vi "LIVE+PSM+SAVING_modified.vi"() -> ()   [LabVIEW 2020]
uses:
  C:/Users/Hannah/Documents/GitHub/pan-ASLM/LabVIEW camera PVCam/Dependencies/PVCamNET.dll
  Dependencies/PVCamNET.dll
panel:
  out "Min  2":u32
  out "Max 2":u32
  out "RawImageData 3":u16[](array[numeric])
  out "SavingPath":string="C:\\Users\\Hannah\\Downloads\\Parameters\\"
  in  "Path":path=path "C:/Users/Hannah/Downloads/Parameters"
  in  "exposure resolution":enum16{"milliseconds", "Microseconds"}(ring)
  out "Saving":bool
  out "Capturing":bool
  in  "seq_save":bool
  in  "seq_start":bool
  in  "FramesToCapture":u16
  in  "Full CCD Height":u16=3200
  in  "Full CCD Width":u16=3200
  in  "Full CCD":bool
  in  "Get ROI":bool
  in  "Height":u16=3192
  in  "Y":u16=4
  in  "Width":u16=416
  in  "X":u16=1452
  out "Trigger Mode":i32=2304
  in  "Trigger In Behaviour":string(combo)="Internal Trigger"
  out "Exp. out":i32
  in  "Trigger Out Behaviour":string(combo)="First Row"
  out "Boolean":bool
  in  "Scan Direction Reset":bool
  out "Scan Line Time":dbl=7063.0 format="%#_14g"
  in  "Scan Width":dbl
  in  "Scan Line Delay":dbl=2.0
  in  "Scan Direction":string(combo)="Down"
  in  "Scan Mode":string(combo)="Auto"
  in  "Exposure Time":dbl=10.0
  in  "Live":bool
  in  "Camera Status":bool
  in  "Uninit":bool
  in  "Live stop":bool
  in  "Live start":bool
  in  "Open":bool
  # "Do not press the red LabVIEW circular button – this will not properly close the camera."
  # "Description:\nThis interface can be used for both live imaging\nand sequence acquisition.\n\nSteps to run:\n1. Click the \"Run\" arrow\n2. Click \"Open\"\n3. Add desired parameters\n\nTo run live imaging: click \"Live Start\". If\nparameters need to be changed while imaging,\nfirst click \"Live Stop\" and then change\nparameters before starting again.\n\nTo execute sequence acquisition: click\n\"Sequence Start\". AFTER sequence has been\ncompleted (signified by the \"Capturing\" light\nturning off), click \"Sequence Save\" to save\nimages to desired folder.\n\n4. Click \"Close\" after finished imaging"
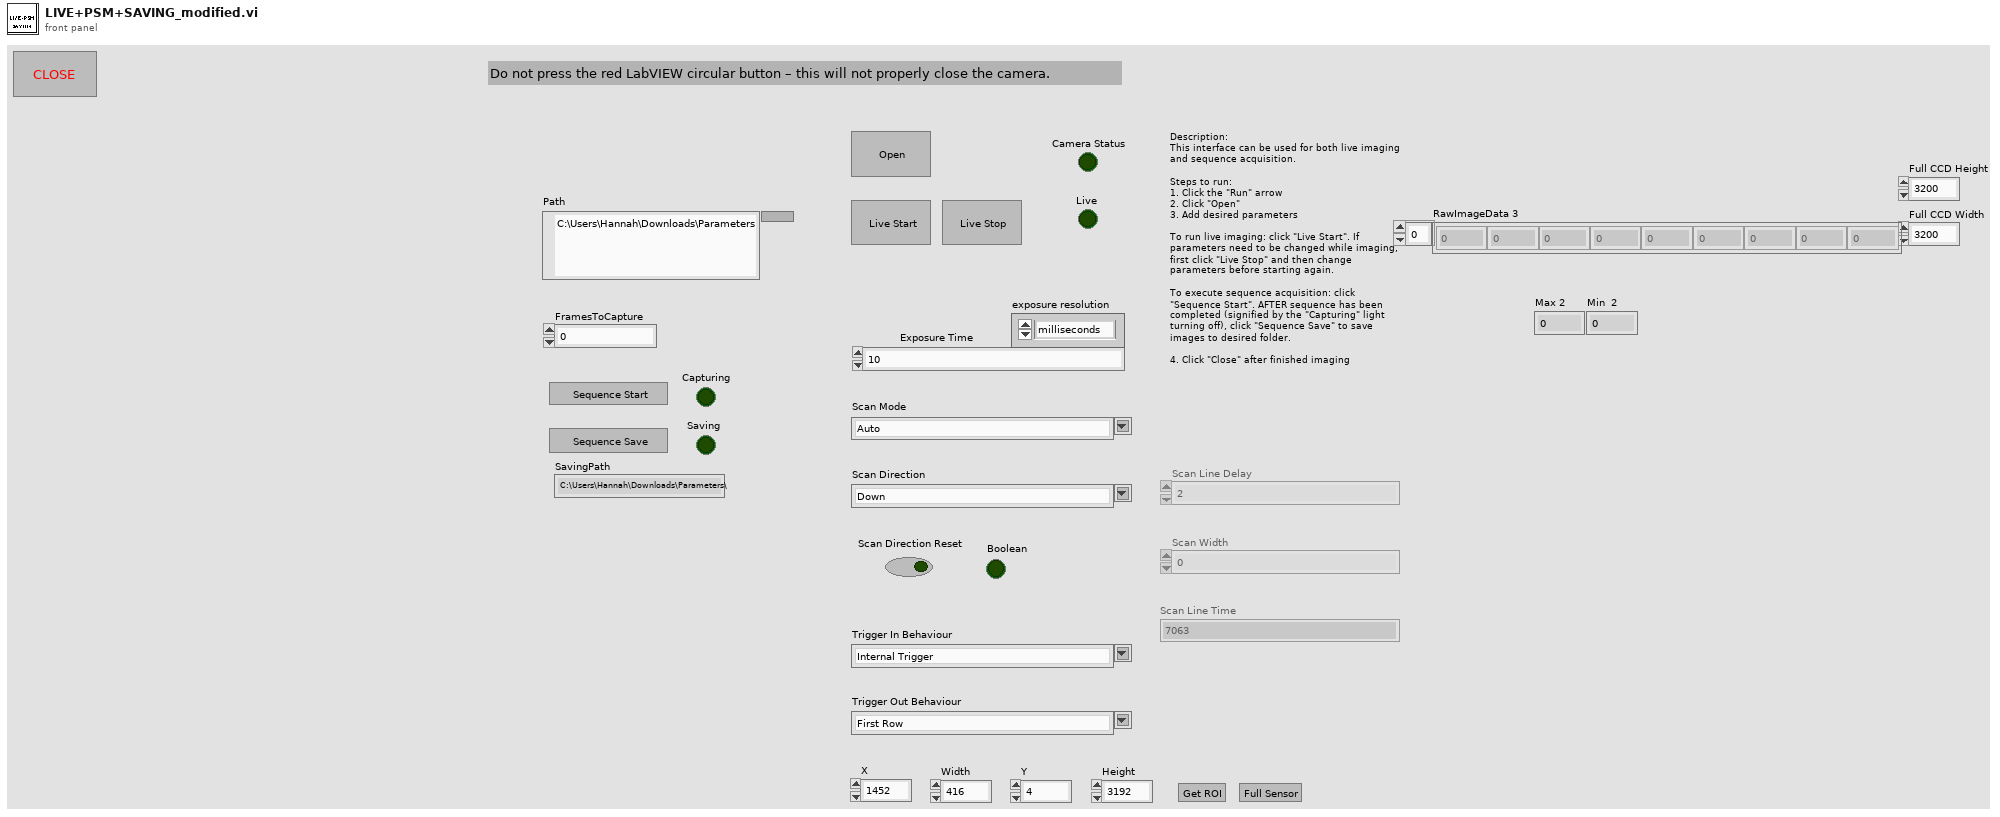
[diagram p1: front panel]
types:
  T1 = enum8{"Enabled", "Disabled", "Disabled and Grayed Out"}
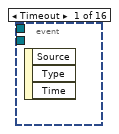
[diagram p2: hidden frame]
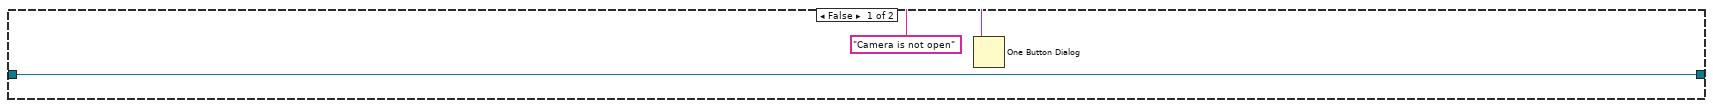
[diagram p14: hidden frame]
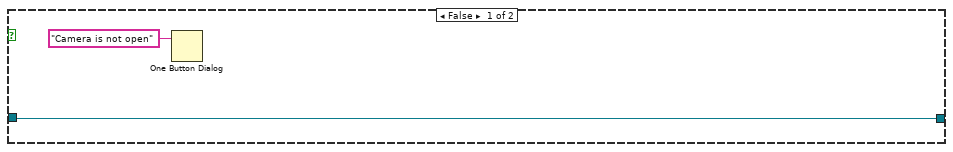
[diagram p19: hidden frame]
diagram:
  w20 = T1."Disabled and Grayed Out" ("Disabled")
  n1 = flat-sequence {
    tunnel: [w34] -> w33
    tunnel: w33 -> [w36]
    tunnel: [w35] -> w32
    tunnel: w32 -> [w844]
    frame #0 {
      n2 = property class="Library"() -> ("Instance"=w34:refnum<k24>)  [unwired: 2 in, 2 out]
    }
    frame #1 {
      n3 = while {
        tunnel: w36 -> [w41]
        shift-right: [w40] -> _
        shift-left: _ -> [w38]
        tunnel: [w39] -> w35
        stop <- w37 stop-if-true
        n4 = event shown="[2] \"seq_start\": Value Change" {
          selector: _ -> [_ _ _ _ _ _ _ _ _ _ _ _ _ _ _ _]
          dyn-events: _ -> [_ _ _ _ _ _ _ _ _ _ _ _ _ _ _ _]
          timeout: _ -> [_ _ _ _ _ _ _ _ _ _ _ _ _ _ _ _]
          tunnel: w41 -> [_ w46 _ _ _ _ _ _ w530 _ _ _ _ w766 _ w817]
          tunnel: [_ w45 w186 w225 w253 w280 w417 w480 w531 w600 w637 w706 w730 w767 w794 w818] -> w40
          tunnel: [_ w44 _ _ _ _ _ _ w530 _ _ _ _ w766 _ w817] -> w39
          tunnel: w38 -> [_ w43 w187 w224 w255 w281 w410 w470 w532 w601 w638 w707 w731 w768 w795 w819]
          tunnel: [_ _ _ _ _ _ _ _ _ _ _ _ _ _ _ w816] -> w37
          event Timeout {
            n5 = event-data() -> ()  [unwired: 1 in, 3 out]
          }
          event "Open": Value Change {
            n6 = event-data() -> ()  [unwired: 1 in, 6 out]
            n7 = case shown="True" "Open" {
              tunnel: w46 -> [w48 w54]
              tunnel: [w47 w53] -> w45
              tunnel: [w48 w52] -> w44
              tunnel: w43 -> [w47 w49]
              frame False {
              }
              frame True {
                n8 = local read "Camera Status"() -> (w51:bool)
                n9 = Not(x=w51) -> (.not. x?=w50:bool)
                n10 = case shown="True" w50 {
                  tunnel: w54 -> [w55 w61]
                  tunnel: [w56 w60] -> w53
                  tunnel: [w55 w57] -> w52
                  tunnel: w49 -> [w56 _]
                  frame False {
                  }
                  frame True {
                    n11 = flat-sequence {
                      tunnel: w61 -> [w66]
                      tunnel: [w68] -> w63
                      tunnel: [w67] -> w62
                      tunnel: w63 -> [w74]
                      tunnel: w62 -> [w75]
                      tunnel: [w75] -> w59
                      tunnel: [w73] -> w58
                      tunnel: [w76] -> w57
                      tunnel: [w78] -> w60
                      tunnel: w59 -> [w114]
                      tunnel: w58 -> [w76]
                      frame #0 {
                        # "Getting Camera at 0 index"
                        n12 = property class="Library"(reference=w66) -> ("Instance"=w65:refnum<k24>)  [unwired: 1 in, 2 out]
                        n13 = invoke class="Library" method="LoadCameras"(reference=w65) -> (reference out=w64:refnum<k24>)  [unwired: 2 in, 2 out]
                        n14 = property class="Library"(reference=w64) -> (reference out=w68:refnum<k24>, "Cameras"=w71:refnum<k24>)  [unwired: 1 in, 1 out]
                        n15 = invoke class="PmReadOnlyObservableCollection`" method="get_Item"(reference=w71, "index"=0) -> ("get_Item"=w69:refnum<k24>)  [unwired: 2 in, 3 out]
                        n16 = invoke class="Camera" method="Open"(reference=w69) -> (reference out=w67:refnum<k24>)  [unwired: 2 in, 2 out]
                      }
                      frame #1 {
                        n17 = invoke class="Library" method="ShowImage"(reference=w74, "cam"=w75) -> (reference out=w73:refnum<k24>)  [unwired: 2 in, 3 out]
                        n18 = local write "Camera Status"(TRUE ("Camera Status")) -> ()
                      }
                      frame #2 {
                        # "register callback"
                        n19 = local read "Exposure Time"() -> (w86:dbl)
                        n20 = property class="Camera"(reference=w114) -> (reference out=w97:refnum<k24>, "Settings"=w87:refnum<k24>)  [unwired: 1 in, 1 out]
                        n21 = property class="CameraSettings"(reference=w87) -> ("ScanMode"=w113:refnum<k24>, "ScanDirection"=w109:refnum<k24>, "ScanLineDelay"=w104:refnum<k24>, "ScanWidth"=w93:refnum<k24>, "ScanLineTime"=w85:refnum<k24>, "ScanDirectionReset"=w100:refnum<k24>, "ExposeOutMode"=w89:refnum<k24>, "SensorHeight"=w80:refnum<k24>, "SensorWidth"=w79:refnum<k24>)  [unwired: 1 in, 2 out]
                        n22 = property class="CameraSettings"(reference=w87, "Exposure"=w86) -> ()  [unwired: 1 in, 2 out]
                        n23 = property class="Camera"(reference=w97) -> (reference out=w78:refnum<k24>, "AcquisitionBuffer"=w96:refnum<k24>)  [unwired: 1 in, 1 out]
                        n24 = property class="AcqBuffer"(reference=w96, "UseScaling"=TRUE) -> ()  [unwired: 1 in, 2 out]
                        n25 = property class="PmNumericParam`1[[System.UInt32"(reference=w80) -> ("Max"=w82:u32)  [unwired: 1 in, 2 out]
                        n26 = property class="PmNumericParam`1[[System.UInt32"(reference=w79) -> ("Max"=w81:u32)  [unwired: 1 in, 2 out]
                        n27 = property class="PmNumericParam`1[[System.Int64,"(reference=w85) -> (reference out=w83:refnum<k24>, "Available"=w84:bool)  [unwired: 1 in, 1 out]
                        n28 = property class="PmEnumParam"(reference=w109) -> (reference out=w107:refnum<k24>, "Available"=w108:bool)  [unwired: 1 in, 1 out]
                        n29 = property class="PmEnumParam"(reference=w113) -> (reference out=w111:refnum<k24>, "Available"=w112:bool)  [unwired: 1 in, 1 out]
                        n30 = property class="PmBoolParam"(reference=w100) -> (reference out=w98:refnum<k24>, "Available"=w99:bool)  [unwired: 1 in, 1 out]
                        n31 = property class="PmEnumParam"(reference=w89) -> (reference out=w90:refnum<k24>, "Available"=w91:bool)  [unwired: 1 in, 1 out]
                        n32 = control-ref of="Trigger Out Behaviour"() -> (w88:refnum<vi>)
                        n33 = control-ref of="Scan Mode"() -> (w110:refnum<vi>)
                        n34 = control-ref of="Scan Direction"() -> (w106:refnum<vi>)
                        n35 = control-ref of="Scan Line Time"() -> (w101:refnum<vi>)
                        n36 = local write "Full CCD Width"(w81) -> ()
                        n37 = local write "Full CCD Height"(w82) -> ()
                        n38 = case shown="True" w108 {
                          tunnel: w107 -> [_ w163]
                          tunnel: w106 -> [_ w154]
                          frame False {
                          }
                          frame True {
                            n39 = property class="PmEnumParam"(reference=w163) -> (reference out=w153:refnum<k24>, "Options"=w162:refnum<k24>)  [unwired: 1 in, 1 out]
                            n40 = property class="PmReadOnlyObservableCollection`"(reference=w162) -> (reference out=w160:refnum<k24>, "Count"=w161:i32)  [unwired: 1 in, 1 out]
                            n41 = for {
                              N: w161 -> [_]
                              tunnel: w160 -> [w168]
                              tunnel: [w165] -> w157
                              tunnel: [w164] -> w156 mode=indexing
                              i -> [w167]
                              n42 = invoke class="PmReadOnlyObservableCollection`" method="get_Item"(reference=w168, "index"=w167) -> (reference out=w165:refnum<k24>, "get_Item"=w166:refnum<k24>)  [unwired: 2 in, 2 out]
                              n43 = property class="PmEnumItem"(reference=w166) -> ("Name"=w164:string)  [unwired: 1 in, 2 out]
                            }
                            n44 = invoke class="PmReadOnlyObservableCollection`" method="get_Item"(reference=w157, "index"=0) -> ("get_Item"=w158:refnum<k24>)  [unwired: 2 in, 3 out]
                            n45 = property class="PmEnumItem"(reference=w158) -> (reference out=w152:refnum<k24>, "Name"=w155:string)  [unwired: 1 in, 1 out]
                            n46 = property class="PmEnumParam"(reference=w153, "Current"=w152) -> ()  [unwired: 1 in, 2 out]
                            n47 = property class="CmbBox"(reference=w154, "Strings[]"=w156, "Value"=w155) -> ()  [unwired: 1 in, 2 out]
                          }
                        }
                        n48 = case shown="True" w112 {
                          tunnel: w111 -> [_ w180]
                          tunnel: w110 -> [_ w173]
                          frame False {
                          }
                          frame True {
                            n49 = property class="PmEnumParam"(reference=w180) -> (reference out=w172:refnum<k24>, "Options"=w179:refnum<k24>)  [unwired: 1 in, 1 out]
                            n50 = property class="PmReadOnlyObservableCollection`"(reference=w179) -> (reference out=w177:refnum<k24>, "Count"=w178:i32)  [unwired: 1 in, 1 out]
                            n51 = for {
                              N: w178 -> [_]
                              tunnel: w177 -> [w185]
                              tunnel: [w182] -> w169
                              tunnel: [w181] -> w175 mode=indexing
                              i -> [w184]
                              n52 = invoke class="PmReadOnlyObservableCollection`" method="get_Item"(reference=w185, "index"=w184) -> (reference out=w182:refnum<k24>, "get_Item"=w183:refnum<k24>)  [unwired: 2 in, 2 out]
                              n53 = property class="PmEnumItem"(reference=w183) -> ("Name"=w181:string)  [unwired: 1 in, 2 out]
                            }
                            n54 = invoke class="PmReadOnlyObservableCollection`" method="get_Item"(reference=w169, "index"=0) -> ("get_Item"=w171:refnum<k24>)  [unwired: 2 in, 3 out]
                            n55 = property class="PmEnumItem"(reference=w171) -> (reference out=w170:refnum<k24>, "Name"=w174:string)  [unwired: 1 in, 1 out]
                            n56 = property class="PmEnumParam"(reference=w172, "Current"=w170) -> ()  [unwired: 1 in, 2 out]
                            n57 = property class="CmbBox"(reference=w173, "Strings[]"=w175, "Value"=w174) -> ()  [unwired: 1 in, 2 out]
                          }
                        }
                        n58 = property class="PmNumericParam`1[[System.UInt32"(reference=w104) -> (reference out=w102:refnum<k24>, "Available"=w103:bool)  [unwired: 1 in, 1 out]
                        n59 = case shown="True" w99 {
                          tunnel: w98 -> [_ w131]
                          frame False {
                          }
                          frame True {
                            n60 = property class="PmBoolParam"(reference=w131) -> ("Current"=w130:bool)  [unwired: 1 in, 2 out]
                            n61 = local write "Scan Direction Reset"(w130) -> ()
                          }
                        }
                        n62 = case shown="True" w91 {
                          tunnel: w90 -> [_ w124]
                          tunnel: w88 -> [_ w115]
                          frame False {
                          }
                          frame True {
                            n63 = property class="PmEnumParam"(reference=w124) -> ("Options"=w123:refnum<k24>)  [unwired: 1 in, 2 out]
                            n64 = property class="PmReadOnlyObservableCollection`"(reference=w123) -> (reference out=w121:refnum<k24>, "Count"=w122:i32)  [unwired: 1 in, 1 out]
                            n65 = for {
                              N: w122 -> [_]
                              tunnel: w121 -> [w129]
                              tunnel: [w127] -> w118
                              tunnel: [w126] -> w117 mode=indexing
                              i -> [w125]
                              n66 = invoke class="PmReadOnlyObservableCollection`" method="get_Item"(reference=w129, "index"=w125) -> (reference out=w127:refnum<k24>, "get_Item"=w128:refnum<k24>)  [unwired: 2 in, 2 out]
                              n67 = property class="PmEnumItem"(reference=w128) -> ("Name"=w126:string)  [unwired: 1 in, 2 out]
                            }
                            n68 = invoke class="PmReadOnlyObservableCollection`" method="get_Item"(reference=w118, "index"=0) -> ("get_Item"=w119:refnum<k24>)  [unwired: 2 in, 3 out]
                            n69 = property class="PmEnumItem"(reference=w119) -> ("Name"=w116:string)  [unwired: 1 in, 2 out]
                            n70 = property class="CmbBox"(reference=w115, "Strings[]"=w117, "Value"=w116) -> ()  [unwired: 1 in, 2 out]
                          }
                        }
                        n71 = property class="PmNumericParam`1[[System.UInt32"(reference=w93) -> (reference out=w92:refnum<k24>, "Available"=w94:bool)  [unwired: 1 in, 1 out]
                        n72 = case shown="True" w84 {
                          tunnel: w101 -> [_ w133]
                          tunnel: w83 -> [_ w132]
                          frame False {
                          }
                          frame True {
                            n73 = property class="PmNumericParam`1[[System.Int64,"(reference=w132) -> ("Max"=w134:i64, "Min"=w135:i64, "Current"=w136:i64)  [unwired: 1 in, 2 out]
                            n74 = In Range and Coerce(upper limit=w134, x=w136, lower limit=w135) -> (coerced(x)=w137:i64)  [unwired: 1 out]
                            n75 = property class="DigNum (strict)"(reference=w133, "Value"=w137) -> ()  [unwired: 1 in, 2 out]
                          }
                        }
                        n76 = control-ref of="Scan Width"() -> (w105:refnum<vi>)
                        n77 = control-ref of="Scan Line Delay"() -> (w77:refnum<vi>)
                        n78 = case shown="True" w103 {
                          tunnel: w105 -> [_ w145]
                          tunnel: w102 -> [_ w148]
                          frame False {
                          }
                          frame True {
                            n79 = property class="PmNumericParam`1[[System.UInt32"(reference=w148) -> (reference out=w147:refnum<k24>, "Max"=w149:u32, "Min"=w150:u32, "Current"=w151:u32)  [unwired: 1 in, 1 out]
                            n80 = In Range and Coerce(upper limit=w149, x=w151, lower limit=w150) -> (coerced(x)=w146:u32)  [unwired: 1 out]
                            n81 = property class="PmNumericParam`1[[System.UInt32"(reference=w147, "Current"=w146) -> ()  [unwired: 1 in, 2 out]
                            n82 = property class="DigNum (strict)"(reference=w145, "Value"=w146) -> ()  [unwired: 1 in, 2 out]
                          }
                        }
                        n83 = case shown="True" w94 {
                          tunnel: w77 -> [_ w138]
                          tunnel: w92 -> [_ w141]
                          frame False {
                          }
                          frame True {
                            n84 = property class="PmNumericParam`1[[System.UInt32"(reference=w141) -> (reference out=w140:refnum<k24>, "Max"=w142:u32, "Min"=w143:u32, "Current"=w144:u32)  [unwired: 1 in, 1 out]
                            n85 = In Range and Coerce(upper limit=w142, x=w144, lower limit=w143) -> (coerced(x)=w139:u32)  [unwired: 1 out]
                            n86 = property class="PmNumericParam`1[[System.UInt32"(reference=w140, "Current"=w139) -> ()  [unwired: 1 in, 2 out]
                            n87 = property class="DigNum (strict)"(reference=w138, "Value"=w139) -> ()  [unwired: 1 in, 2 out]
                          }
                        }
                      }
                    }
                  }
                }
              }
            }
          }
          event "seq_start": Value Change {
            n88 = event-data() -> ()  [unwired: 1 in, 6 out]
            n89 = case shown="True" "seq_start" {
              tunnel: w187 -> [w189 w192]
              tunnel: [w189 w190] -> w186
              frame False {
              }
              frame True {
                n90 = local read "Camera Status"() -> (w191:bool)
                n91 = case shown="True" w191 {
                  tunnel: w192 -> [w193 w200]
                  tunnel: [w193 w198] -> w190
                  frame False {
                    n92 = One Button Dialog(message="Camera is not open") -> ()  [unwired: 1 in, 1 out]
                  }
                  frame True {
                    w201 = 0 items=["Idle", "Capturing"] ("Status")
                    n93 = property class="Camera"(reference=w200) -> (reference out=w199:refnum<k24>, "IsOpen"=w195:bool, "Status"=w202:i32)  [unwired: 1 in, 1 out]
                    n94 = Equal?(x=w202, y=w201) -> (x = y?=w196:bool)
                    n95 = And(x=w195, y=w196) -> (x .and. y?=w197:bool)
                    n96 = case shown="True" w197 {
                      tunnel: w199 -> [w203 w206]
                      tunnel: [w203 w205] -> w198
                      frame False {
                      }
                      frame True {
                        n97 = flat-sequence {
                          tunnel: w206 -> [w208]
                          tunnel: [w207] -> w204
                          tunnel: [w214] -> w205
                          tunnel: w204 -> [w222]
                          frame #0 {
                            n98 = property class="Camera" props=["Settings", "AcquisitionBuffer"](reference=w208) -> (reference out=w207:refnum<k24>)  [unwired: 1 in, 3 out]
                            n99 = disable-structure shown="Disabled" {
                              disable-tunnel: w207 -> [w209 _]
                              frame Disabled {
                                # "Register a callback to know the camera's state \n(eg. idle, capturing)"
                                n100 = control-ref of="Capturing"() -> (w210:refnum<vi>)
                                n101 = vi-ref "PropertyChangedEventCallbackForCameraState.vi"() -> ("vi reference"=w211:refnum<vi>)
                                n102 = node(w209, w211, w210) -> ()  [unwired: 2 in, 2 out]
                              }
                              frame Enabled {
                              }
                            }
                          }
                          frame #1 {
                            w212 = u16 10 ("FramesToCapture")
                            n103 = invoke class="Camera" method="StartSequence"(reference=w222) -> (reference out=w215:refnum<k24>)  [unwired: 2 in, 2 out]
                            n104 = property class="Camera"(reference=w215) -> (reference out=w214:refnum<k24>, "Settings"=w216:refnum<k24>, "AcquisitionBuffer"=w217:refnum<k24>)  [unwired: 1 in, 1 out]
                            n105 = property class="CameraSettings"(reference=w216, "FramesToCapture"=w212) -> ()  [unwired: 1 in, 2 out]
                            n106 = property class="AcqBuffer"(reference=w217, "BufferSize"=w212) -> ("FrameToDisplay"=w213:refnum<k24>)  [unwired: 1 in, 2 out]
                            n107 = property class="Frame"(reference=w213) -> (reference out=w218:refnum<k24>, "Max"=→"Max 2":u32, "Min"=→"Min  2":u32, "RawImageData"=→"RawImageData 3":u16[])  [unwired: 1 in, 1 out]
                            n108 = Close Reference(reference=w218) -> ()  [unwired: 1 in, 1 out]
                          }
                        }
                      }
                    }
                  }
                }
              }
            }
          }
          event "seq_save": Value Change {
            n109 = event-data() -> ()  [unwired: 1 in, 6 out]
            n110 = case shown="True" "seq_save" {
              tunnel: [w226 w228] -> w225
              tunnel: w224 -> [w226 w227]
              frame False {
              }
              frame True {
                n111 = local read "Camera Status"() -> (w229:bool)
                n112 = case shown="True" w229 {
                  tunnel: [w230 w236] -> w228
                  tunnel: w227 -> [w230 w235]
                  frame False {
                    n113 = One Button Dialog(message="Camera is not open") -> ()  [unwired: 1 in, 1 out]
                  }
                  frame True {
                    w238 = 0 items=["Idle", "Capturing"] ("Status")
                    n114 = property class="Camera"(reference=w235) -> (reference out=w237:refnum<k24>, "IsOpen"=w233:bool, "Status"=w239:i32)  [unwired: 1 in, 1 out]
                    n115 = Equal?(x=w239, y=w238) -> (x = y?=w232:bool)
                    n116 = And(x=w233, y=w232) -> (x .and. y?=w234:bool)
                    n117 = case shown="True" w234 {
                      tunnel: w237 -> [w240 w243]
                      tunnel: [w240 w242] -> w236
                      frame False {
                      }
                      frame True {
                        n118 = flat-sequence {
                          tunnel: [w245] -> w241
                          tunnel: w243 -> [w244]
                          tunnel: [w248] -> w242
                          tunnel: w241 -> [w248]
                          frame #0 {
                            # "Save all the frames in the buffer to a Tiff image"
                            n119 = property class="Camera"(reference=w244) -> (reference out=w245:refnum<k24>, "AcquisitionBuffer"=w247:refnum<k24>)  [unwired: 1 in, 1 out]
                            n120 = local write "Saving"(TRUE ("Camera Status")) -> ()
                            n121 = invoke class="AcqBuffer" method="SaveAsTiff"(reference=w247) -> ()  [unwired: 2 in, 3 out]
                          }
                          frame #1 {
                            n122 = local write "Saving"(FALSE ("Camera Status")) -> ()
                          }
                        }
                      }
                    }
                  }
                }
              }
            }
          }
          event "Scan Direction": Value Change {
            w256 = 0 items=["Idle", "Capturing"] ("Status")
            n123 = event-data() -> ()  [unwired: 1 in, 6 out]
            n124 = property class="Camera"(reference=w255) -> (reference out=w254:refnum<k24>, "IsOpen"=w250:bool, "Status"=w257:i32)  [unwired: 1 in, 1 out]
            n125 = Equal?(x=w257, y=w256) -> (x = y?=w251:bool)
            n126 = And(x=w250, y=w251) -> (x .and. y?=w252:bool)
            n127 = case shown="True" w252 {
              tunnel: w254 -> [w258 w262]
              tunnel: [w258 w259] -> w253
              frame False {
              }
              frame True {
                n128 = property class="Camera"(reference=w262) -> (reference out=w259:refnum<k24>, "Settings"=w263:refnum<k24>)  [unwired: 1 in, 1 out]
                n129 = property class="CameraSettings"(reference=w263) -> ("ScanDirection"=w261:refnum<k24>)  [unwired: 1 in, 2 out]
                n130 = property class="PmEnumParam"(reference=w261) -> (reference out=w264:refnum<k24>, "Available"=w265:bool)  [unwired: 1 in, 1 out]
                n131 = control-ref of="Scan Mode"() -> (w260:refnum<vi>)
                n132 = case shown="True" w265 {
                  tunnel: w264 -> [_ w273]
                  tunnel: w260 -> [_ w267]
                  frame False {
                  }
                  frame True {
                    n133 = property class="CmbBox"(reference=w267) -> (reference out=w269:refnum<vi>, "Strings[]"=w274:string[])  [unwired: 1 in, 1 out]
                    n134 = property class="CmbBox"(reference=w269) -> ("Value"=w268:string)  [unwired: 1 in, 2 out]
                    n135 = while {
                      tunnel: w274 -> [w278] mode=indexing
                      tunnel: [w276] -> _
                      tunnel: w268 -> [w275]
                      i -> [w276]
                      stop <- w277 stop-if-true
                      n136 = Equal?(x=w278, y=w275) -> (x = y?=w277:bool)
                    }
                    n137 = property class="PmEnumParam"(reference=w273) -> (reference out=w271:refnum<k24>, "Options"=w272:refnum<k24>)  [unwired: 1 in, 1 out]
                    n138 = invoke class="PmReadOnlyObservableCollection`" method="get_Item"(reference=w272, "index"=1) -> ("get_Item"=w270:refnum<k24>)  [unwired: 2 in, 3 out]
                    n139 = property class="PmEnumParam"(reference=w271, "Current"=w270) -> ()  [unwired: 1 in, 2 out]
                  }
                }
              }
            }
          }
          event "Scan Mode", "Scan Direction Reset": Value Change {
            n140 = event-data() -> ()  [unwired: 1 in, 6 out]
            n141 = local read "Camera Status"() -> (w279:bool)
            n142 = case shown="True" w279 {
              tunnel: w281 -> [w282 w284]
              tunnel: [w282 w291] -> w280
              frame False {
                n143 = One Button Dialog(message="Camera is not open") -> ()  [unwired: 1 in, 1 out]
              }
              frame True {
                w289 = 0 items=["Idle", "Capturing"] ("Status")
                n144 = property class="Camera"(reference=w284) -> (reference out=w286:refnum<k24>, "IsOpen"=w287:bool, "Status"=w290:i32)  [unwired: 1 in, 1 out]
                n145 = Equal?(x=w290, y=w289) -> (x = y?=w288:bool)
                n146 = And(x=w287, y=w288) -> (x .and. y?=w285:bool)
                n147 = case shown="True" w285 {
                  tunnel: w286 -> [w292 w331]
                  tunnel: [w292 w326] -> w291
                  frame False {
                  }
                  frame True {
                    # "For Scan mode type if Auto is chosen then Scan Width and Scan Line Delay are not configurable.\nIf Line Delay is chosen then Scan Line is configurable, but Scan Width is not configurable.\nSimilarly if Scan Delay is chosen then Scan Line Delay is configurable, but Scan Width is not configurable."
                    n148 = property class="Camera"(reference=w331) -> (reference out=w326:refnum<k24>, "Settings"=w330:refnum<k24>)  [unwired: 1 in, 1 out]
                    n149 = property class="CameraSettings"(reference=w330) -> (error out=w323:errorcluster, "ScanMode"=w329:refnum<k24>, "ScanDirection"=w325:refnum<k24>, "ScanWidth"=w321:refnum<k24>, "ScanLineDelay"=w320:refnum<k24>, "ScanLineTime"=w309:refnum<k24>, "ScanDirectionReset"=w298:refnum<k24>)  [unwired: 1 in, 1 out]
                    n150 = property class="PmEnumParam"(reference=w329, error in=w323) -> (reference out=w327:refnum<k24>, error out=w324:errorcluster, "Available"=w328:bool)
                    n151 = control-ref of="Scan Mode"() -> (w322:refnum<vi>)
                    n152 = case shown="True" w328 {
                      tunnel: w327 -> [_ w404]
                      tunnel: w322 -> [_ w399]
                      tunnel: w324 -> [w392 w398]
                      tunnel: [w392 w393] -> w308
                      frame False {
                      }
                      frame True {
                        n153 = property class="CmbBox"(reference=w399) -> (reference out=w400:refnum<vi>, "Strings[]"=w405:string[])  [unwired: 1 in, 1 out]
                        n154 = property class="PmEnumParam"(reference=w404, error in=w398) -> (reference out=w401:refnum<k24>, error out=w397:errorcluster, "Options"=w403:refnum<k24>)
                        n155 = property class="CmbBox"(reference=w400) -> ("Value"=w395:string)  [unwired: 1 in, 2 out]
                        n156 = while {
                          tunnel: w405 -> [w409] mode=indexing
                          tunnel: [w407] -> w402
                          tunnel: w395 -> [w406]
                          i -> [w407]
                          stop <- w408 stop-if-true
                          n157 = Equal?(x=w409, y=w406) -> (x = y?=w408:bool)
                        }
                        n158 = invoke class="PmReadOnlyObservableCollection`" method="get_Item"(reference=w403, error in=w397, "index"=w402) -> (error out=w396:errorcluster, "get_Item"=w394:refnum<k24>)  [unwired: 1 in, 2 out]
                        n159 = property class="PmEnumParam" props=["Current", "IsReadOnly"](reference=w401, error in=w396, "Current"=w394) -> (error out=w393:errorcluster)  [unwired: 2 out]
                      }
                    }
                    n160 = property class="PmEnumParam"(reference=w325, error in=w308) -> (reference out=w317:refnum<k24>, error out=w311:errorcluster, "Available"=w318:bool)
                    n161 = control-ref of="Scan Direction"() -> (w319:refnum<vi>)
                    n162 = case shown="True" w318 {
                      tunnel: w317 -> [_ w386]
                      tunnel: w319 -> [_ w378]
                      tunnel: w311 -> [w370 w377]
                      tunnel: [w370 w371] -> w310
                      frame False {
                      }
                      frame True {
                        n163 = property class="PmEnumParam"(reference=w386, error in=w377) -> (reference out=w372:refnum<k24>, error out=w376:errorcluster, "Options"=w385:refnum<k24>)
                        n164 = property class="PmReadOnlyObservableCollection`"(reference=w385) -> (reference out=w383:refnum<k24>, "Count"=w384:i32)  [unwired: 1 in, 1 out]
                        n165 = for {
                          N: w384 -> [_]
                          tunnel: w383 -> [w391]
                          tunnel: [w388] -> w381
                          tunnel: [w387] -> w380 mode=indexing
                          i -> [w390]
                          n166 = invoke class="PmReadOnlyObservableCollection`" method="get_Item"(reference=w391, "index"=w390) -> (reference out=w388:refnum<k24>, "get_Item"=w389:refnum<k24>)  [unwired: 2 in, 2 out]
                          n167 = property class="PmEnumItem"(reference=w389) -> ("Name"=w387:string)  [unwired: 1 in, 2 out]
                        }
                        n168 = invoke class="PmReadOnlyObservableCollection`" method="get_Item"(reference=w381, error in=w376, "index"=0) -> (error out=w375:errorcluster, "get_Item"=w373:refnum<k24>)  [unwired: 1 in, 2 out]
                        n169 = property class="PmEnumParam"(reference=w372, "Current"=w373) -> ()  [unwired: 1 in, 2 out]
                        n170 = property class="PmEnumItem"(reference=w373, error in=w375) -> (error out=w374:errorcluster, "Name"=w379:string)  [unwired: 1 out]
                        n171 = property class="CmbBox"(reference=w378, error in=w374, "Strings[]"=w380, "Value"=w379) -> (error out=w371:errorcluster)  [unwired: 1 out]
                      }
                    }
                    n172 = property class="PmNumericParam`1[[System.UInt32"(reference=w321, error in=w310) -> (reference out=w314:refnum<k24>, error out=w313:errorcluster, "Available"=w315:bool)
                    n173 = control-ref of="Scan Width"() -> (w316:refnum<vi>)
                    n174 = case shown="True" w315 {
                      tunnel: w316 -> [_ w366]
                      tunnel: w314 -> [_ w363]
                      tunnel: w313 -> [w360 w365]
                      tunnel: [w360 w364] -> w312
                      frame False {
                      }
                      frame True {
                        n175 = property class="PmNumericParam`1[[System.UInt32"(reference=w363) -> ("Current"=w367:u32, "IsReadOnly"=w362:bool)  [unwired: 1 in, 2 out]
                        n176 = case shown="False" w362 {
                          tunnel: [T1."Enabled" ("Disabled") T1."Disabled and Grayed Out" ("Disabled")] -> w361
                          frame False {
                          }
                          frame True {
                          }
                        }
                        n177 = property class="DigNum (strict)"(reference=w366, error in=w365, "Value"=w367, "DisabledEnum"=w361) -> (error out=w364:errorcluster)  [unwired: 1 out]
                      }
                    }
                    n178 = property class="PmNumericParam`1[[System.UInt32"(reference=w320, error in=w312) -> (reference out=w305:refnum<k24>, error out=w299:errorcluster, "Available"=w306:bool)
                    n179 = control-ref of="Scan Line Delay"() -> (w300:refnum<vi>)
                    n180 = case shown="True" w306 {
                      tunnel: w300 -> [_ w356]
                      tunnel: w305 -> [_ w353]
                      tunnel: w299 -> [w350 w355]
                      tunnel: [w350 w354] -> w302
                      frame False {
                      }
                      frame True {
                        n181 = property class="PmNumericParam`1[[System.UInt32"(reference=w353) -> ("Current"=w357:u32, "IsReadOnly"=w352:bool)  [unwired: 1 in, 2 out]
                        n182 = case shown="False" w352 {
                          tunnel: [T1."Enabled" ("Disabled") T1."Disabled and Grayed Out" ("Disabled")] -> w351
                          frame False {
                          }
                          frame True {
                          }
                        }
                        n183 = property class="DigNum (strict)"(reference=w356, error in=w355, "Value"=w357, "DisabledEnum"=w351) -> (error out=w354:errorcluster)  [unwired: 1 out]
                      }
                    }
                    n184 = property class="PmNumericParam`1[[System.Int64,"(reference=w309, error in=w302) -> (reference out=w304:refnum<k24>, error out=w301:errorcluster, "Available"=w307:bool)
                    n185 = control-ref of="Scan Line Time"() -> (w303:refnum<vi>)
                    n186 = case shown="True" w307 {
                      tunnel: w303 -> [_ w346]
                      tunnel: w304 -> [_ w343]
                      tunnel: w301 -> [w340 w345]
                      tunnel: [w340 w344] -> w294
                      frame False {
                      }
                      frame True {
                        n187 = property class="PmNumericParam`1[[System.Int64,"(reference=w343) -> ("Current"=w347:i64, "IsReadOnly"=w342:bool)  [unwired: 1 in, 2 out]
                        n188 = case shown="True" w342 {
                          tunnel: [T1."Enabled" ("Disabled") T1."Disabled and Grayed Out" ("Disabled")] -> w341
                          frame False {
                          }
                          frame True {
                          }
                        }
                        n189 = property class="DigNum (strict)"(reference=w346, error in=w345, "Value"=w347, "DisabledEnum"=w341) -> (error out=w344:errorcluster)  [unwired: 1 out]
                      }
                    }
                    n190 = property class="PmBoolParam"(reference=w298, error in=w294) -> (reference out=w296:refnum<k24>, error out=w293:errorcluster, "Available"=w297:bool)
                    n191 = control-ref of="Scan Direction Reset"() -> (w295:refnum<vi>)
                    n192 = case shown="True" w297 {
                      tunnel: w296 -> [_ w337]
                      tunnel: w295 -> [_ w339]
                      tunnel: w293 -> [_ w334]
                      frame False {
                      }
                      frame True {
                        n193 = property class="Bool (strict)"(reference=w339, error in=w334) -> (error out=w333:errorcluster, "Value"=w338:bool)  [unwired: 1 out]
                        n194 = property class="PmBoolParam"(reference=w337, error in=w333, "Current"=w338) -> (reference out=w336:refnum<k24>, error out=w332:errorcluster)
                        n195 = property class="PmBoolParam"(reference=w336, error in=w332) -> ("Current"=w335:bool)  [unwired: 2 out]
                        n196 = local write "Boolean"(w335) -> ()
                      }
                    }
                  }
                }
              }
            }
          }
          event "Scan Line Delay": Value Change {
            w415 = 0 items=["Idle", "Capturing"] ("Status")
            n197 = event-data() -> ()  [unwired: 1 in, 6 out]
            n198 = property class="Camera"(reference=w410) -> (reference out=w412:refnum<k24>, "IsOpen"=w413:bool, "Status"=w416:i32)  [unwired: 1 in, 1 out]
            n199 = Equal?(x=w416, y=w415) -> (x = y?=w414:bool)
            n200 = control-ref of="Scan Line Delay"() -> (w419:refnum<vi>)
            n201 = control-ref of="Scan Width"() -> (w420:refnum<vi>)
            n202 = control-ref of="Scan Line Time"() -> (w418:refnum<vi>)
            n203 = And(x=w413, y=w414) -> (x .and. y?=w411:bool)
            n204 = case shown="True" w411 {
              tunnel: w412 -> [w421 w443]
              tunnel: [w421 w442] -> w417
              tunnel: w419 -> [_ w441]
              tunnel: w420 -> [_ w440]
              tunnel: w418 -> [_ w424]
              frame False {
              }
              frame True {
                n205 = property class="Camera"(reference=w443) -> (reference out=w442:refnum<k24>, "Settings"=w439:refnum<k24>)  [unwired: 1 in, 1 out]
                n206 = property class="CameraSettings"(reference=w439) -> (reference out=w429:refnum<k24>, error out=w435:errorcluster, "ScanLineDelay"=w438:refnum<k24>)  [unwired: 1 in]
                n207 = property class="PmNumericParam`1[[System.UInt32"(reference=w438, error in=w435) -> (reference out=w436:refnum<k24>, error out=w434:errorcluster, "Available"=w437:bool)
                n208 = case shown="True" w437 {
                  tunnel: w441 -> [_ w461]
                  tunnel: w436 -> [_ w460]
                  tunnel: w434 -> [w456 w459]
                  tunnel: [w456 w457] -> w430
                  frame False {
                  }
                  frame True {
                    n209 = property class="PmNumericParam`1[[System.UInt32"(reference=w460) -> (reference out=w464:refnum<k24>, "Max"=w462:u32, "Min"=w463:u32)  [unwired: 1 in, 1 out]
                    n210 = property class="DigNum (strict)"(reference=w461, error in=w459) -> (reference out=w468:refnum<vi>, error out=w458:errorcluster, "Value"=w467:dbl)
                    n211 = In Range and Coerce(upper limit=w462, x=w467, lower limit=w463) -> (coerced(x)=w466:dbl)  [unwired: 1 out]
                    n212 = property class="PmNumericParam`1[[System.UInt32"(reference=w464, "Current"=w466) -> (reference out=w465:refnum<k24>)  [unwired: 1 in, 1 out]
                    n213 = property class="PmNumericParam`1[[System.UInt32"(reference=w465) -> ("Current"=w469:u32)  [unwired: 1 in, 2 out]
                    n214 = property class="DigNum (strict)"(reference=w468, error in=w458, "Value"=w469) -> (error out=w457:errorcluster)  [unwired: 1 out]
                  }
                }
                n215 = property class="CameraSettings"(reference=w429) -> ("ScanWidth"=w428:refnum<k24>, "ScanLineTime"=w427:refnum<k24>)  [unwired: 1 in, 2 out]
                n216 = property class="PmNumericParam`1[[System.UInt32"(reference=w428, error in=w430) -> (reference out=w432:refnum<k24>, error out=w431:errorcluster, "Available"=w433:bool)
                n217 = case shown="True" w433 {
                  tunnel: w440 -> [_ w453]
                  tunnel: w432 -> [_ w455]
                  tunnel: w431 -> [w449 w451]
                  tunnel: [w449 w454] -> w423
                  frame False {
                  }
                  frame True {
                    n218 = property class="PmNumericParam`1[[System.UInt32"(reference=w455, error in=w451) -> (error out=w450:errorcluster, "Current"=w452:u32)  [unwired: 1 out]
                    n219 = property class="DigNum (strict)"(reference=w453, error in=w450, "Value"=w452) -> (error out=w454:errorcluster)  [unwired: 1 out]
                  }
                }
                n220 = property class="PmNumericParam`1[[System.Int64,"(reference=w427, error in=w423) -> (reference out=w425:refnum<k24>, error out=w422:errorcluster, "Available"=w426:bool)
                n221 = case shown="True" w426 {
                  tunnel: w425 -> [_ w448]
                  tunnel: w424 -> [_ w446]
                  tunnel: w422 -> [_ w445]
                  frame False {
                  }
                  frame True {
                    n222 = property class="PmNumericParam`1[[System.Int64,"(reference=w448, error in=w445) -> (error out=w444:errorcluster, "Current"=w447:i64)  [unwired: 1 out]
                    n223 = property class="DigNum (strict)"(reference=w446, error in=w444, "Value"=w447) -> ()  [unwired: 2 out]
                  }
                }
              }
            }
          }
          event "Scan Width": Value Change {
            w475 = 0 items=["Idle", "Capturing"] ("Status")
            n224 = event-data() -> ()  [unwired: 1 in, 6 out]
            n225 = property class="Camera"(reference=w470) -> (reference out=w472:refnum<k24>, "IsOpen"=w473:bool, "Status"=w476:i32)  [unwired: 1 in, 1 out]
            n226 = Equal?(x=w476, y=w475) -> (x = y?=w474:bool)
            n227 = control-ref of="Scan Line Delay"() -> (w478:refnum<vi>)
            n228 = control-ref of="Scan Line Time"() -> (w477:refnum<vi>)
            n229 = control-ref of="Scan Width"() -> (w479:refnum<vi>)
            n230 = And(x=w473, y=w474) -> (x .and. y?=w471:bool)
            n231 = case shown="True" w471 {
              tunnel: w472 -> [w481 w503]
              tunnel: [w481 w502] -> w480
              tunnel: w479 -> [_ w501]
              tunnel: w478 -> [_ w500]
              tunnel: w477 -> [_ w485]
              frame False {
              }
              frame True {
                n232 = property class="Camera"(reference=w503) -> (reference out=w502:refnum<k24>, "Settings"=w499:refnum<k24>)  [unwired: 1 in, 1 out]
                n233 = property class="CameraSettings"(reference=w499) -> (reference out=w482:refnum<k24>, error out=w495:errorcluster, "ScanWidth"=w498:refnum<k24>)  [unwired: 1 in]
                n234 = property class="PmNumericParam`1[[System.UInt32"(reference=w498, error in=w495) -> (reference out=w496:refnum<k24>, error out=w494:errorcluster, "Available"=w497:bool)
                n235 = case shown="True" w497 {
                  tunnel: w501 -> [_ w520]
                  tunnel: w496 -> [_ w519]
                  tunnel: w494 -> [w515 w518]
                  tunnel: [w515 w516] -> w490
                  frame False {
                  }
                  frame True {
                    n236 = property class="PmNumericParam`1[[System.UInt32"(reference=w519) -> (reference out=w523:refnum<k24>, "Max"=w521:u32, "Min"=w522:u32)  [unwired: 1 in, 1 out]
                    n237 = property class="DigNum (strict)"(reference=w520, error in=w518) -> (reference out=w527:refnum<vi>, error out=w517:errorcluster, "Value"=w526:dbl)
                    n238 = In Range and Coerce(upper limit=w521, x=w526, lower limit=w522) -> (coerced(x)=w525:dbl)  [unwired: 1 out]
                    n239 = property class="PmNumericParam`1[[System.UInt32"(reference=w523, "Current"=w525) -> (reference out=w524:refnum<k24>)  [unwired: 1 in, 1 out]
                    n240 = property class="PmNumericParam`1[[System.UInt32"(reference=w524) -> ("Current"=w528:u32)  [unwired: 1 in, 2 out]
                    n241 = property class="DigNum (strict)"(reference=w527, error in=w517, "Value"=w528) -> (error out=w516:errorcluster)  [unwired: 1 out]
                  }
                }
                n242 = property class="CameraSettings"(reference=w482) -> ("ScanLineDelay"=w489:refnum<k24>, "ScanLineTime"=w488:refnum<k24>)  [unwired: 1 in, 2 out]
                n243 = property class="PmNumericParam`1[[System.UInt32"(reference=w489, error in=w490) -> (reference out=w492:refnum<k24>, error out=w491:errorcluster, "Available"=w493:bool)
                n244 = case shown="True" w493 {
                  tunnel: w500 -> [_ w511]
                  tunnel: w492 -> [_ w514]
                  tunnel: w491 -> [w509 w512]
                  tunnel: [w509 w513] -> w484
                  frame False {
                  }
                  frame True {
                    n245 = property class="PmNumericParam`1[[System.UInt32"(reference=w514) -> ("Current"=w510:u32)  [unwired: 1 in, 2 out]
                    n246 = property class="DigNum (strict)"(reference=w511, error in=w512, "Value"=w510) -> (error out=w513:errorcluster)  [unwired: 1 out]
                  }
                }
                n247 = property class="PmNumericParam`1[[System.Int64,"(reference=w488, error in=w484) -> (reference out=w486:refnum<k24>, error out=w483:errorcluster, "Available"=w487:bool)
                n248 = case shown="True" w487 {
                  tunnel: w486 -> [_ w508]
                  tunnel: w485 -> [_ w506]
                  tunnel: w483 -> [_ w505]
                  frame False {
                  }
                  frame True {
                    n249 = property class="PmNumericParam`1[[System.Int64,"(reference=w508, error in=w505) -> (error out=w504:errorcluster, "Current"=w507:i64)  [unwired: 1 out]
                    n250 = property class="DigNum (strict)"(reference=w506, error in=w504, "Value"=w507) -> ()  [unwired: 2 out]
                  }
                }
              }
            }
          }
          event "Trigger In Behaviour", "Trigger Out Behaviour": Value Change {
            n251 = event-data() -> ()  [unwired: 1 in, 6 out]
            n252 = local read "Camera Status"() -> (w529:bool)
            n253 = case shown="True" w529 {
              tunnel: w532 -> [w534 w538]
              tunnel: [w534 w535] -> w531
              frame False {
                n254 = One Button Dialog(message="Camera is not open") -> ()  [unwired: 1 in, 1 out]
              }
              frame True {
                w543 = 0 items=["Idle", "Capturing"] ("Status")
                n255 = property class="Camera"(reference=w538) -> (reference out=w536:refnum<k24>, "IsOpen"=w542:bool, "Status"=w544:i32)  [unwired: 1 in, 1 out]
                n256 = Equal?(x=w542, y=TRUE) -> (x = y?=w540:bool)
                n257 = Equal?(x=w544, y=w543) -> (x = y?=w539:bool)
                n258 = Equal?(x=w540, y=w539) -> (x = y?=w537:bool)
                n259 = case shown="True" w537 {
                  tunnel: w536 -> [w545 w569]
                  tunnel: [w545 w561] -> w535
                  frame False {
                  }
                  frame True {
                    n260 = property class="Camera"(reference=w569) -> (reference out=w561:refnum<k24>, "Settings"=w548:refnum<k24>)  [unwired: 1 in, 1 out]
                    n261 = local read "exposure resolution"() -> (w546:enum16{"milliseconds", "Microseconds"})
                    n262 = property class="CameraSettings"(reference=w548) -> (reference out=w556:refnum<k24>, "ExposureTime"=w555:refnum<k24>, "ExposureMode"=w549:refnum<k24>, "ExposeOutMode"=w554:refnum<k24>, "ExpResIndex"=w547:refnum<k24>)  [unwired: 1 in, 1 out]
                    n263 = property class="PmNumericParam`1[[System.UInt32"(reference=w547, "Current"=w546) -> ()  [unwired: 1 in, 2 out]
                    n264 = property class="PmNumericParam`1[[System.UInt64"(reference=w555) -> (reference out=w566:refnum<k24>, "Max"=w568:u64, "Min"=w567:u64)  [unwired: 1 in, 1 out]
                    n265 = property class="PmEnumParam"(reference=w549) -> (reference out=w551:refnum<k24>, "Available"=w550:bool)  [unwired: 1 in, 1 out]
                    n266 = property class="PmEnumParam"(reference=w554) -> (reference out=w559:refnum<k24>, "Available"=w560:bool)  [unwired: 1 in, 1 out]
                    n267 = control-ref of="Trigger In Behaviour"() -> (w552:refnum<vi>)
                    n268 = local read "Exposure Time"() -> (w563:dbl)
                    n269 = control-ref of="Trigger Mode"() -> (w553:refnum<vi>)
                    n270 = case shown="True" w550 {
                      tunnel: w551 -> [_ w579]
                      tunnel: w553 -> [_ w573]
                      tunnel: w552 -> [_ w570]
                      frame False {
                      }
                      frame True {
                        n271 = property class="CmbBox"(reference=w570) -> (reference out=w572:refnum<vi>, "Strings[]"=w580:string[])  [unwired: 1 in, 1 out]
                        n272 = property class="CmbBox"(reference=w572) -> ("Value"=w571:string)  [unwired: 1 in, 2 out]
                        n273 = while {
                          tunnel: w580 -> [w584] mode=indexing
                          tunnel: [w582] -> w577
                          tunnel: w571 -> [w581]
                          i -> [w582]
                          stop <- w583 stop-if-true
                          n274 = Equal?(x=w584, y=w581) -> (x = y?=w583:bool)
                        }
                        n275 = property class="PmEnumParam"(reference=w579) -> (reference out=w576:refnum<k24>, "Options"=w578:refnum<k24>)  [unwired: 1 in, 1 out]
                        n276 = invoke class="PmReadOnlyObservableCollection`" method="get_Item"(reference=w578, "index"=w577) -> ("get_Item"=w575:refnum<k24>)  [unwired: 2 in, 3 out]
                        n277 = property class="PmEnumParam"(reference=w576, "Current"=w575) -> ()  [unwired: 1 in, 2 out]
                        n278 = property class="PmEnumItem"(reference=w575) -> ("Value"=w574:i32)  [unwired: 1 in, 2 out]
                        n279 = property class="DigNum (strict)"(reference=w573, "Value"=w574) -> ()  [unwired: 1 in, 2 out]
                      }
                    }
                    n280 = In Range and Coerce(upper limit=w568, x=w563, lower limit=w567) -> (coerced(x)=w564:dbl)  [unwired: 1 out]
                    n281 = control-ref of="Trigger Out Behaviour"() -> (w557:refnum<vi>)
                    n282 = control-ref of="Exp. out"() -> (w558:refnum<vi>)
                    n283 = property class="CameraSettings"(reference=w556, "Exposure"=w564) -> ()  [unwired: 1 in, 2 out]
                    n284 = property class="PmNumericParam`1[[System.UInt64"(reference=w566, "Current"=w564) -> (reference out=w565:refnum<k24>)  [unwired: 1 in, 1 out]
                    n285 = case shown="True" w560 {
                      tunnel: w559 -> [_ w594]
                      tunnel: w558 -> [_ w588]
                      tunnel: w557 -> [_ w585]
                      frame False {
                      }
                      frame True {
                        n286 = property class="CmbBox"(reference=w585) -> (reference out=w587:refnum<vi>, "Strings[]"=w595:string[])  [unwired: 1 in, 1 out]
                        n287 = property class="CmbBox"(reference=w587) -> ("Value"=w586:string)  [unwired: 1 in, 2 out]
                        n288 = while {
                          tunnel: w595 -> [w599] mode=indexing
                          tunnel: [w597] -> w592
                          tunnel: w586 -> [w596]
                          i -> [w597]
                          stop <- w598 stop-if-true
                          n289 = Equal?(x=w599, y=w596) -> (x = y?=w598:bool)
                        }
                        n290 = property class="PmEnumParam"(reference=w594) -> (reference out=w591:refnum<k24>, "Options"=w593:refnum<k24>)  [unwired: 1 in, 1 out]
                        n291 = invoke class="PmReadOnlyObservableCollection`" method="get_Item"(reference=w593, "index"=w592) -> ("get_Item"=w590:refnum<k24>)  [unwired: 2 in, 3 out]
                        n292 = property class="PmEnumParam"(reference=w591, "Current"=w590) -> ()  [unwired: 1 in, 2 out]
                        n293 = property class="PmEnumItem"(reference=w590) -> ("Value"=w589:i32)  [unwired: 1 in, 2 out]
                        n294 = property class="DigNum (strict)"(reference=w588, "Value"=w589) -> ()  [unwired: 1 in, 2 out]
                      }
                    }
                    n295 = property class="PmNumericParam`1[[System.UInt64"(reference=w565) -> ("Current"=w562:u64)  [unwired: 1 in, 2 out]
                    n296 = local write "Exposure Time"(w562) -> ()
                  }
                }
              }
            }
          }
          event "Get ROI": Value Change {
            n297 = event-data() -> ()  [unwired: 1 in, 6 out]
            n298 = case shown="True" "Get ROI" {
              tunnel: w601 -> [w603 w606]
              tunnel: [w603 w605] -> w600
              frame False {
              }
              frame True {
                n299 = local read "Camera Status"() -> (w604:bool)
                n300 = case shown="True" w604 {
                  tunnel: w606 -> [w608 w612]
                  tunnel: [w608 w609] -> w605
                  frame False {
                    n301 = One Button Dialog(message="Camera is not open") -> ()  [unwired: 1 in, 1 out]
                  }
                  frame True {
                    w617 = 0 items=["Idle", "Capturing"] ("Status")
                    n302 = property class="Camera"(reference=w612) -> (reference out=w611:refnum<k24>, "IsOpen"=w616:bool, "Status"=w618:i32)  [unwired: 1 in, 1 out]
                    n303 = Equal?(x=w618, y=w617) -> (x = y?=w613:bool)
                    n304 = Equal?(x=w616, y=TRUE) -> (x = y?=w614:bool)
                    n305 = Equal?(x=w614, y=w613) -> (x = y?=w610:bool)
                    n306 = case shown="True" w610 {
                      tunnel: w611 -> [w620 w628]
                      tunnel: [w620 w627] -> w609
                      frame False {
                        n307 = One Button Dialog(message="Camera must be idle.") -> ()  [unwired: 1 in, 1 out]
                      }
                      frame True {
                        n308 = property class="Camera"(reference=w628) -> (reference out=w627:refnum<k24>, "Settings"=w626:refnum<k24>)  [unwired: 1 in, 1 out]
                        n309 = property class="CameraSettings"(reference=w626) -> ("Regions"=w625:refnum<k24>)  [unwired: 1 in, 2 out]
                        n310 = property class="PmObservableCollection`1[[PVCam"(reference=w625) -> (reference out=w621:refnum<k24>, "Count"=w624:i32)  [unwired: 1 in, 1 out]
                        n311 = Greater?(x=w624, y=0) -> (0:w622:bool)
                        n312 = case shown="True" w622 {
                          tunnel: w621 -> [_ w630]
                          frame False {
                            n313 = One Button Dialog(message="ROI is not created.") -> ()  [unwired: 1 in, 1 out]
                          }
                          frame True {
                            n314 = invoke class="PmObservableCollection`1[[PVCam" method="get_Item"(reference=w630, "index"=0) -> ("get_Item"=w636:refnum<k24>)  [unwired: 2 in, 3 out]
                            n315 = property class="PmRegion"(reference=w636) -> ("Height"=w634:u16, "Width"=w633:u16, "X"=w632:u16, "Y"=w631:u16)  [unwired: 1 in, 2 out]
                            n316 = local write "Width"(w633) -> ()
                            n317 = local write "X"(w632) -> ()
                            n318 = local write "Y"(w631) -> ()
                            n319 = local write "Height"(w634) -> ()
                          }
                        }
                      }
                    }
                  }
                }
              }
            }
          }
          event "X", "Width", "Y", "Height": Value Change {
            n320 = event-data() -> ()  [unwired: 1 in, 6 out]
            n321 = local read "Camera Status"() -> (w639:bool)
            n322 = case shown="True" w639 {
              tunnel: w638 -> [w640 w646]
              tunnel: [w640 w644] -> w637
              frame False {
              }
              frame True {
                w647 = 0 items=["Idle", "Capturing"] ("Status")
                n323 = property class="Camera"(reference=w646) -> (reference out=w645:refnum<k24>, "IsOpen"=w642:bool, "Status"=w648:i32)  [unwired: 1 in, 1 out]
                n324 = Equal?(x=w648, y=w647) -> (x = y?=w643:bool)
                n325 = And(x=w642, y=w643) -> (x .and. y?=w641:bool)
                n326 = case shown="True" w641 {
                  tunnel: w645 -> [w649 w651]
                  tunnel: [w649 w652] -> w644
                  frame False {
                  }
                  frame True {
                    n327 = flat-sequence {
                      tunnel: w651 -> [w653]
                      tunnel: [w653] -> w650
                      tunnel: [w697] -> w652
                      tunnel: w650 -> [w690]
                      frame #0 {
                        # "if (!( x >= 0\n            && (x+width) <= full_width\n            &&  0 < width \n            && y >= 0\n            && (y+height) <= full_height\n            && 0 < height ))\n        {\n           printf(\"Incorrect range for a ROI. \\n\");\n        }"
                        n328 = local read "Width"() -> (w676:u16)
                        n329 = local read "Height"() -> (w674:u16)
                        n330 = local read "X"() -> (w677:u16)
                        n331 = local read "Y"() -> (w673:u16)
                        n332 = Add(x=w674, y=w673) -> (x+y=w669:u16)
                        n333 = Add(x=w677, y=w676) -> (x+y=w671:u16)
                        n334 = local read "Full CCD Height"() -> (w670:u16)
                        n335 = local read "Full CCD Width"() -> (w672:u16)
                        n336 = local read "Width"() -> (w668:u16)
                        n337 = local read "Height"() -> (w665:u16)
                        n338 = local read "Y"() -> (w675:u16)
                        n339 = local read "X"() -> (w678:u16)
                        n340 = Greater Or Equal?(x=w675, y=u16 0) -> (x >= y?=w657:bool)
                        n341 = Greater Or Equal?(x=w678, y=u16 0) -> (x >= y?=w660:bool)
                        n342 = Less?(x=u16 0 ("y"), y=w668) -> (x < y?=w658:bool)
                        n343 = Less?(x=u16 0 ("y"), y=w665) -> (x < y?=w655:bool)
                        n344 = Less Or Equal?(x=w671, y=w672) -> (x <= y?=w659:bool)
                        n345 = Less Or Equal?(x=w669, y=w670) -> (x <= y?=w656:bool)
                        n346 = Compound Arithmetic op=AND(w660, w659, w658, w657, w656, w655) -> (w654:bool)
                        n347 = case shown="True" w654 {
                          tunnel: [w682 w689] -> w664
                          tunnel: [u16 0 ("X") w688] -> w661
                          tunnel: [u16 0 ("Y") w687] -> w662
                          tunnel: [w683 w686] -> w663
                          frame False {
                            n348 = local read "Full CCD Height"() -> (w683:u16)
                            n349 = local read "Full CCD Width"() -> (w682:u16)
                            n350 = One Button Dialog(message="Wrong ROI ! Resetting to full CCD") -> ()  [unwired: 1 in, 1 out]
                          }
                          frame True {
                            n351 = local read "Height"() -> (w686:u16)
                            n352 = local read "Width"() -> (w689:u16)
                            n353 = local read "X"() -> (w688:u16)
                            n354 = local read "Y"() -> (w687:u16)
                          }
                        }
                        n355 = local write "Width"(w664) -> ()
                        n356 = local write "Height"(w663) -> ()
                        n357 = local write "X"(w661) -> ()
                        n358 = local write "Y"(w662) -> ()
                      }
                      frame #1 {
                        n359 = property class="Camera"(reference=w690) -> (reference out=w697:refnum<k24>, "Settings"=w696:refnum<k24>)  [unwired: 1 in, 1 out]
                        n360 = property class="CameraSettings"(reference=w696) -> ("Regions"=w695:refnum<k24>)  [unwired: 1 in, 2 out]
                        n361 = property class="PmObservableCollection`1[[PVCam"(reference=w695) -> (reference out=w691:refnum<k24>, "Count"=w694:i32)  [unwired: 1 in, 1 out]
                        n362 = Greater?(x=w694, y=0) -> (0:w692:bool)
                        n363 = case shown="True" w692 {
                          tunnel: w691 -> [_ w703]
                          frame False {
                            n364 = One Button Dialog(message="ROI is not created.") -> ()  [unwired: 1 in, 1 out]
                          }
                          frame True {
                            n365 = invoke class="PmObservableCollection`1[[PVCam" method="get_Item"(reference=w703, "index"=0) -> ("get_Item"=w705:refnum<k24>)  [unwired: 2 in, 3 out]
                            n366 = local read "Height"() -> (w699:u16)
                            n367 = local read "Width"() -> (w702:u16)
                            n368 = local read "X"() -> (w701:u16)
                            n369 = local read "Y"() -> (w700:u16)
                            n370 = property class="PmRegion"(reference=w705, "Height"=w699, "Width"=w702, "X"=w701, "Y"=w700) -> ()  [unwired: 1 in, 2 out]
                          }
                        }
                      }
                    }
                  }
                }
              }
            }
          }
          event "FramesToCapture": Value Change {
            n371 = event-data() -> ()  [unwired: 1 in, 6 out]
            n372 = local read "Camera Status"() -> (w708:bool)
            n373 = case shown="True" w708 {
              tunnel: w707 -> [w709 w715]
              tunnel: [w709 w713] -> w706
              frame False {
              }
              frame True {
                w716 = 0 items=["Idle", "Capturing"] ("Status")
                n374 = property class="Camera"(reference=w715) -> (reference out=w714:refnum<k24>, "IsOpen"=w711:bool, "Status"=w717:i32)  [unwired: 1 in, 1 out]
                n375 = Equal?(x=w717, y=w716) -> (x = y?=w712:bool)
                n376 = And(x=w711, y=w712) -> (x .and. y?=w710:bool)
                n377 = case shown="True" w710 {
                  tunnel: w714 -> [w718 w729]
                  tunnel: [w718 w728] -> w713
                  frame False {
                  }
                  frame True {
                    n378 = Path To String(path="Path") -> (string=w722:string)
                    n379 = property class="Camera"(reference=w729) -> (reference out=w728:refnum<k24>, "Settings"=w726:refnum<k24>, "AcquisitionBuffer"=w727:refnum<k24>)  [unwired: 1 in, 1 out]
                    n380 = Concatenate Strings(w722, "\\" ("string")) -> (w719:string)
                    "SavingPath" <- w719
                    n381 = property class="CameraSettings"(reference=w726, "FramesToCapture"="FramesToCapture") -> ()  [unwired: 1 in, 2 out]
                    n382 = property class="AcqBuffer"(reference=w727, "BufferSize"="FramesToCapture", "BigTiffRequired"=TRUE, "ImageSavingPath"=w719, "MultiPageFrameSize"=u64 1) -> ()  [unwired: 1 in, 2 out]
                  }
                }
              }
            }
          }
          event "Full CCD": Value Change {
            n383 = event-data() -> ()  [unwired: 1 in, 6 out]
            n384 = case shown="True" "Full CCD" {
              tunnel: w731 -> [w733 w736]
              tunnel: [w733 w735] -> w730
              frame False {
              }
              frame True {
                n385 = local read "Camera Status"() -> (w734:bool)
                n386 = case shown="True" w734 {
                  tunnel: w736 -> [w738 w739]
                  tunnel: [w738 w746] -> w735
                  frame False {
                    n387 = One Button Dialog(message="Camera is not open") -> ()  [unwired: 1 in, 1 out]
                  }
                  frame True {
                    w744 = 0 items=["Idle", "Capturing"] ("Status")
                    n388 = property class="Camera"(reference=w739) -> (reference out=w740:refnum<k24>, "IsOpen"=w742:bool, "Status"=w745:i32)  [unwired: 1 in, 1 out]
                    n389 = Equal?(x=w745, y=w744) -> (x = y?=w743:bool)
                    n390 = And(x=w742, y=w743) -> (x .and. y?=w741:bool)
                    n391 = case shown="True" w741 {
                      tunnel: w740 -> [w747 w756]
                      tunnel: [w747 w755] -> w746
                      frame False {
                      }
                      frame True {
                        n392 = property class="Camera"(reference=w756) -> (reference out=w755:refnum<k24>, "Settings"=w754:refnum<k24>)  [unwired: 1 in, 1 out]
                        n393 = property class="CameraSettings"(reference=w754) -> (reference out=w748:refnum<k24>, "Regions"=w749:refnum<k24>)  [unwired: 1 in, 1 out]
                        n394 = property class="PmObservableCollection`1[[PVCam"(reference=w749) -> (reference out=w750:refnum<k24>, "Count"=w753:i32)  [unwired: 1 in, 1 out]
                        n395 = Greater?(x=w753, y=0) -> (0:w751:bool)
                        n396 = case shown="True" w751 {
                          tunnel: w750 -> [_ _]
                          tunnel: w749 -> [_ w765]
                          tunnel: w748 -> [_ w759]
                          frame False {
                          }
                          frame True {
                            n397 = invoke class="PmObservableCollection`1[[PVCam" method="RemoveAt"(reference=w765, "index"=0) -> ()  [unwired: 2 in, 4 out]
                            n398 = property class="CameraSettings"(reference=w759) -> ("SensorWidth"=w761:refnum<k24>)  [unwired: 1 in, 2 out]
                            n399 = property class="CameraSettings"(reference=w759) -> ("SensorHeight"=w762:refnum<k24>)  [unwired: 1 in, 2 out]
                            n400 = property class="PmNumericParam`1[[System.UInt32"(reference=w761) -> ("Current"=w760:u32)  [unwired: 1 in, 2 out]
                            n401 = property class="PmNumericParam`1[[System.UInt32"(reference=w762) -> ("Current"=w763:u32)  [unwired: 1 in, 2 out]
                            n402 = local write "X"(0 ("index")) -> ()
                            n403 = local write "Y"(0 ("index")) -> ()
                            n404 = local write "Width"(w760) -> ()
                            n405 = local write "Height"(w763) -> ()
                          }
                        }
                      }
                    }
                  }
                }
              }
            }
          }
          event "Live start": Value Change {
            n406 = event-data() -> ()  [unwired: 1 in, 6 out]
            n407 = case shown="True" "Live start" {
              tunnel: w768 -> [w770 w773]
              tunnel: [w770 w772] -> w767
              frame False {
              }
              frame True {
                n408 = local read "Camera Status"() -> (w771:bool)
                n409 = case shown="True" w771 {
                  tunnel: w773 -> [w774 w776]
                  tunnel: [w774 w783] -> w772
                  frame False {
                    n410 = One Button Dialog(message="Camera is not open") -> ()  [unwired: 1 in, 1 out]
                  }
                  frame True {
                    w781 = 0 items=["Idle", "Capturing"] ("Status")
                    n411 = property class="Camera"(reference=w776) -> (reference out=w778:refnum<k24>, "IsOpen"=w779:bool, "Status"=w782:i32)  [unwired: 1 in, 1 out]
                    n412 = Equal?(x=w782, y=w781) -> (x = y?=w780:bool)
                    n413 = And(x=w779, y=w780) -> (x .and. y?=w777:bool)
                    n414 = case shown="True" w777 {
                      tunnel: w778 -> [w785 w787]
                      tunnel: [w785 w788] -> w783
                      frame False {
                        n415 = local write "Live"(FALSE ("Live 2")) -> ()
                      }
                      frame True {
                        n416 = flat-sequence {
                          tunnel: w787 -> [w793]
                          tunnel: [w791] -> w786
                          frame #0 {
                            n417 = property class="Camera"(reference=w793) -> (reference out=w791:refnum<k24>, "AcquisitionBuffer"=w790:refnum<k24>)  [unwired: 1 in, 1 out]
                            n418 = property class="AcqBuffer"(reference=w790, "BufferSize"=100) -> ()  [unwired: 1 in, 2 out]
                          }
                        }
                        n419 = local write "Live"(TRUE ("Live")) -> ()
                        n420 = invoke class="Camera" method="StartLive"(reference=w786) -> (reference out=w788:refnum<k24>)  [unwired: 2 in, 2 out]
                      }
                    }
                  }
                }
              }
            }
          }
          event "Live stop": Value Change {
            n421 = event-data() -> ()  [unwired: 1 in, 6 out]
            n422 = case shown="True" "Live stop" {
              tunnel: w795 -> [w797 w800]
              tunnel: [w797 w799] -> w794
              frame False {
              }
              frame True {
                n423 = local read "Camera Status"() -> (w798:bool)
                n424 = case shown="True" w798 {
                  tunnel: w800 -> [w802 w803]
                  tunnel: [w802 w810] -> w799
                  frame False {
                    n425 = One Button Dialog(message="Camera is not open") -> ()  [unwired: 1 in, 1 out]
                  }
                  frame True {
                    w808 = 1 items=["Idle", "Capturing"] ("Status")
                    n426 = property class="Camera"(reference=w803) -> (reference out=w805:refnum<k24>, "IsOpen"=w806:bool, "Status"=w809:i32)  [unwired: 1 in, 1 out]
                    n427 = Equal?(x=w809, y=w808) -> (x = y?=w807:bool)
                    n428 = And(x=w806, y=w807) -> (x .and. y?=w804:bool)
                    n429 = case shown="True" w804 {
                      tunnel: w805 -> [w811 w814]
                      tunnel: [w811 w813] -> w810
                      frame False {
                      }
                      frame True {
                        n430 = invoke class="Camera" method="Stop"(reference=w814) -> (reference out=w813:refnum<k24>)  [unwired: 2 in, 2 out]
                        n431 = local write "Live"(FALSE ("Live 2")) -> ()
                      }
                    }
                  }
                }
              }
            }
          }
          event "Uninit": Value Change {
            n432 = event-data() -> ()  [unwired: 1 in, 6 out]
            n433 = case shown="True" "Uninit" {
              tunnel: w819 -> [w821 w825]
              tunnel: [w821 w824] -> w818
              tunnel: [FALSE ("Camera Status") w822] -> w816
              frame False {
              }
              frame True {
                n434 = local read "Camera Status"() -> (w823:bool)
                n435 = case shown="True" w823 {
                  tunnel: w825 -> [w827 w831]
                  tunnel: [w827 w830] -> w824
                  tunnel: [FALSE ("Camera Status") w829] -> w822
                  frame False {
                  }
                  frame True {
                    n436 = local read "Live"() -> (w828:bool)
                    n437 = case shown="False" w828 {
                      tunnel: w831 -> [w834 w842]
                      tunnel: [w833 w842] -> w830
                      tunnel: [w832 FALSE ("Camera Status")] -> w829
                      frame False {
                        n438 = flat-sequence {
                          tunnel: w834 -> [w837]
                          tunnel: [w836] -> w835
                          tunnel: [w840] -> w833
                          tunnel: w835 -> [w840]
                          tunnel: [TRUE ("Camera Status")] -> w832
                          frame #0 {
                            n439 = invoke class="Camera" method="Close"(reference=w837) -> (reference out=w836:refnum<k24>)  [unwired: 2 in, 2 out]
                          }
                          frame #1 {
                            n440 = local write "Camera Status"(FALSE ("Camera Status")) -> ()
                          }
                        }
                      }
                      frame True {
                      }
                    }
                  }
                }
              }
            }
          }
        }
      }
    }
    frame #2 {
      n441 = invoke class="Library" method="Release"(reference=w844) -> (reference out=w845:refnum<k24>)  [unwired: 2 in, 2 out]
      n442 = Wait (ms)(milliseconds to wait=u32 100) -> ()  [unwired: 1 out]
      n443 = Close Reference(reference=w845) -> ()  [unwired: 1 in, 1 out]
    }
    frame #3 {
      n444 = invoke class="GC" method="Collect"() -> ()  [unwired: 3 in, 3 out]
    }
  }
  n445 = local write "Camera Status"(FALSE ("Camera Status")) -> ()
  n446 = control-ref of="FramesToCapture"() -> (w2:refnum<vi>)
  n447 = property class="DigNum (strict)"(reference=w2, "Value"=10) -> ()  [unwired: 1 in, 2 out]
  n448 = String To Path(string="") -> (path=w5:path)
  n449 = control-ref of="Path"() -> (w3:refnum<vi>)
  n450 = property class="Path"(reference=w3, "Value"=w5) -> ()  [unwired: 1 in, 2 out]
  n451 = control-ref of="Scan Mode"() -> (w30:refnum<vi>)
  n452 = control-ref of="Scan Direction"() -> (w27:refnum<vi>)
  n453 = property class="CmbBox"(reference=w30, "Value"="", "Strings[]"=string[] [] ("Strings []")) -> ()  [unwired: 1 in, 2 out]
  n454 = property class="CmbBox"(reference=w27, "Value"="", "Strings[]"=string[] [] ("Strings []")) -> ()  [unwired: 1 in, 2 out]
  n455 = control-ref of="Trigger Mode"() -> (w11:refnum<vi>)
  n456 = control-ref of="Scan Line Delay"() -> (w23:refnum<vi>)
  n457 = control-ref of="Scan Line Time"() -> (w22:refnum<vi>)
  n458 = control-ref of="Exp. out"() -> (w12:refnum<vi>)
  n459 = control-ref of="Scan Width"() -> (w26:refnum<vi>)
  n460 = control-ref of="Exp. out"() -> (w15:refnum<vi>)
  n461 = property class="DigNum (strict)"(reference=w12, "Visible"=FALSE) -> ()  [unwired: 1 in, 2 out]
  n462 = property class="DigNum (strict)"(reference=w26, "Value"=0.0) -> ()  [unwired: 1 in, 2 out]
  n463 = property class="DigNum (strict)"(reference=w11, "Visible"=FALSE) -> ()  [unwired: 1 in, 2 out]
  n464 = property class="DigNum (strict)"(reference=w15, "Value"=0) -> ()  [unwired: 1 in, 2 out]
  n465 = property class="DigNum (strict)"(reference=w22, "Value"=0.0) -> ()  [unwired: 1 in, 2 out]
  n466 = property class="DigNum (strict)"(reference=w23, "Value"=0.0) -> ()  [unwired: 1 in, 2 out]
  n467 = property on="Scan Width" class="DigNum (strict)"("DisabledEnum"=w20) -> ()  [unwired: 2 in, 2 out]
  n468 = property on="Scan Line Delay" class="DigNum (strict)"("DisabledEnum"=w20) -> ()  [unwired: 2 in, 2 out]
  n469 = control-ref of="exposure resolution"() -> (w7:refnum<vi>)
  n470 = local write "Scan Direction Reset"(FALSE ("Boolean")) -> ()
  n471 = property class="Enum (strict)"(reference=w7, "Value"="exposure resolution") -> ()  [unwired: 1 in, 2 out]
  n472 = control-ref of="Trigger Out Behaviour"() -> (w17:refnum<vi>)
  n473 = property class="CmbBox"(reference=w17, "Value"="") -> ()  [unwired: 1 in, 2 out]
  "Boolean" <- FALSE ("Boolean")
